vi "WPI_CANJaguar_SetPID.vi"(0 "CAN Jaguar Ref":T1={"DeviceStatus"={"status"=FALSE, "code"=0, "source"=""}, "Type"=enum."PWM", "PWM"={"PWM Channel"=enum."PWM 1", "DeadBand"={"Name"="", "maxPositivePwm"=0, "minPositivePwm"=0, "centerPwm"=0, "maxNegativePwm"=0, "minNegativePwm"=0, "angularRange"=0}}, "CAN"={"Device Number"=0, "Control Mode"=enum."Percent VBus", "Semaphore"=refnum, "Max Vout"=12.0, "TalonSRX Control Mode"=enum."Percent VBus"}, "Invert"=FALSE}, 5 "P":dbl, 7 "I":dbl, 9 "D":dbl, 11 "error in (no error)":errorcluster) -> (4 "CAN Jaguar Ref":T1={"DeviceStatus"={"status"=FALSE, "code"=0, "source"=""}, "Type"=enum."PWM", "PWM"={"PWM Channel"=enum."PWM 1", "DeadBand"={"Name"="", "maxPositivePwm"=0, "minPositivePwm"=0, "centerPwm"=0, "maxNegativePwm"=0, "minNegativePwm"=0, "angularRange"=0}}, "CAN"={"Device Number"=0, "Control Mode"=enum."Percent VBus", "Semaphore"=refnum, "Max Vout"=12.0, "TalonSRX Control Mode"=enum."Percent VBus"}, "Invert"=FALSE}, 15 "error out":errorcluster)   [LabVIEW 2016]
doc: "Set the PID constants that should be used by the active controller on the Jaguar.\n\nThis VI only applies in <B>Current</B>, <B>Position</B>, and <B>Speed</B> modes."
uses:
  <vilib>/Rock Robotics/WPI/MotorControl/WPI_MotorControlDeviceRef.ctl
  <vilib>/Rock Robotics/WPI/MotorControl/WPI_MotorControlType.ctl
  <vilib>/Rock Robotics/SystemInterfaces/DIO/FPGA_DIOPWMChannel.ctl
  <vilib>/Rock Robotics/WPI/PWM/WPI_PWMDeadband.ctl
  <vilib>/Rock Robotics/WPI/CAN/Jaguar/SubVIs/WPI_CANJaguar_ControlMode.ctl
  <vilib>/Rock Robotics/WPI/CAN/TalonSRX/WPI_CANTalonSRX_APIControlMode.ctl
  <vilib>/Rock Robotics/WPI/CAN/Jaguar/SubVIs/WPI_CAN_MotorMessageIDs.ctl
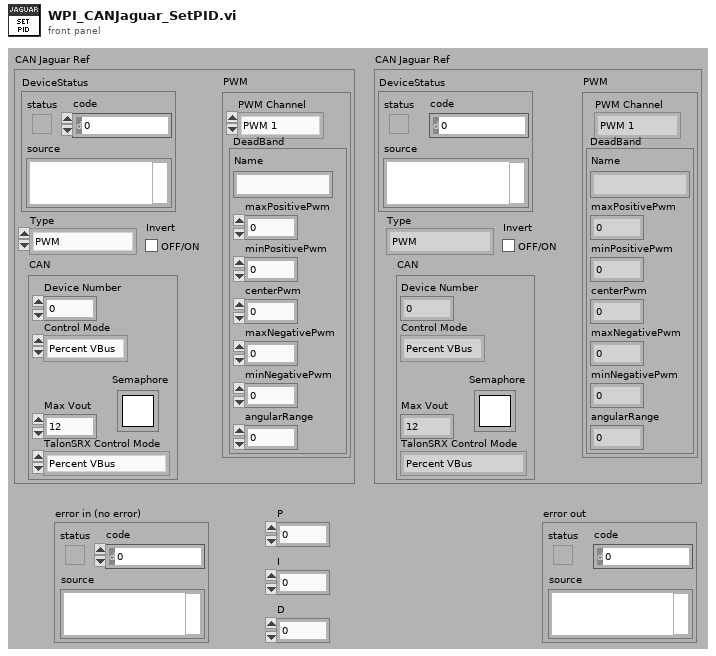
[diagram p1: front panel]
types:
  T1 = typedef "WPI_MotorControlDeviceRef.ctl" = cluster{"DeviceStatus":errorcluster, "Type":T2, "PWM":cluster{"PWM Channel":T3, "DeadBand":T4}, "CAN":cluster{"Device Number":u8, "Control Mode":T5, "Semaphore":T6, "Max Vout":dbl, "TalonSRX Control Mode":T7}, "Invert":bool}
  T2 = typedef "WPI_MotorControlType.ctl" = enum16{"PWM", "CAN", "CANTalonSRX"}
  T3 = typedef "FPGA_DIOPWMChannel.ctl" = enum8{"PWM 0", "PWM 1", "PWM 2", "PWM 3", "PWM 4", "PWM 5", "PWM 6", "PWM 7", "PWM 8", "PWM 9", "PWM MXP 0", "PWM MXP 1", "PWM MXP 2", "PWM MXP 3", "PWM MXP 4", "PWM MXP 5", "PWM MXP 6", "PWM MXP 7", "PWM MXP 8", "PWM MXP 9", "Invalid"}
  T4 = typedef "WPI_PWMDeadband.ctl" = cluster{"Name":string, "maxPositivePwm":i32, "minPositivePwm":i32, "centerPwm":i32, "maxNegativePwm":i32, "minNegativePwm":i32, "angularRange":u16}
  T5 = typedef "WPI_CANJaguar_ControlMode.ctl" = enum8{"Percent VBus", "Current", "Speed", "Position", "Voltage"}
  T6 = typedef "Semaphore RefNum" = refnum<k1>
  T7 = typedef "WPI_CANTalonSRX_APIControlMode.ctl" = enum8{"Percent VBus", "Speed", "Position", "Slave", "Unchanged / Invalid", "Voltage Compensation", "Current", "Motion Profile"}
  T8 = enum16{"big-endian, network order", "native, host order", "little-endian"}
  T9 = typedef "WPI_CAN_MotorMessageIDs.ctl" = u32
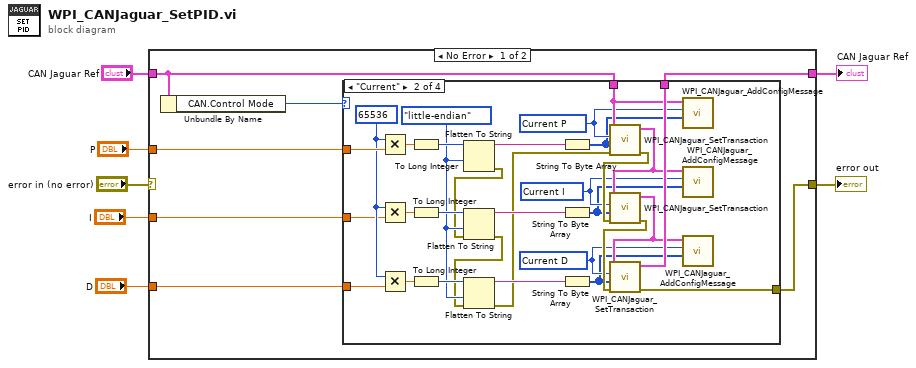
[diagram p0: block diagram]
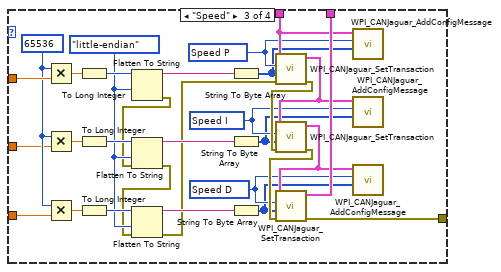
[diagram p3: hidden frame]
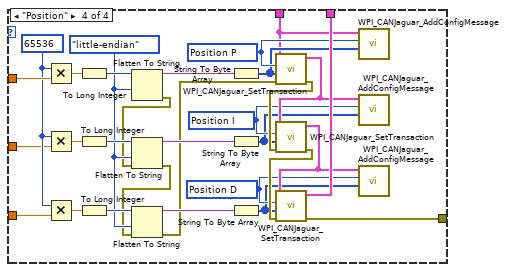
[diagram p4: hidden frame]
diagram:
  n1 = case shown="No Error" "error in (no error)" {
    selector: "error in (no error)" -> [_ w106]
    tunnel: [w11 w106] -> w7
    tunnel: [w8 w107] -> w5
    tunnel: "CAN Jaguar Ref" -> [w9 w107]
    tunnel: "P" -> [w14 _]
    tunnel: "D" -> [w13 _]
    tunnel: "I" -> [w12 _]
    frame No Error {
      n2 = Unbundle By Name(w9) -> ("CAN.Control Mode"=w10:T5)
      n3 = case shown="\"Current\"" w10 {
        tunnel: w14 -> [_ w43 w73 w103]
        tunnel: w13 -> [_ w33 w63 w93]
        tunnel: w12 -> [_ w32 w62 w92]
        tunnel: [_ w27 w58 w88] -> w11
        tunnel: w9 -> [w15 w24 w54 w82]
        tunnel: [w15 w28 w57 w87] -> w8
        frame Default {
        }
        frame "Current" {
          w35 = T8."little-endian" ("byte order (0:big-endian, network order)")
          w17 = T9 33689920 items=["Volt Enable"=33685504, "Volt Disable"=33685568, "Volt Set"=33685632, "Volt Set Ramp"=33685696, "Speed Enable"=33686528, "Speed Disable"=33686592, "Speed Set"=33686656, "Speed P"=33686720, "Speed I"=33686784, "Speed D"=33686848, "Speed Ref"=33686912, "Volt Comp Enable"=33687552, "Volt Comp Disable"=33687616, "Volt Comp Set"=33687680, "Volt Comp In Ramp"=33687744, "Volt Comp Comp Ramp"=33687808, "Position Enable"=33688576, "Position Disable"=33688640, "Position Set"=33688704, "Position P"=33688768, "Position I"=33688832, "Position D"=33688896, "Position Ref"=33688960, "Current Enable"=33689600, "Current Disable"=33689664, "Current Set"=33689728, "Current P"=33689792, "Current I"=33689856, "Current D"=33689920, "Status Percent VBus"=33690624, "Status VBus"=33690688, "Status Current"=33690752, "Status Temp"=33690816, "Status Position"=33690880, "Status Speed"=33690944, "Status Limit"=33691008, "Status Fault"=33691072, "Status Power"=33691136, "Status Control Mode"=33691200, "Status VOut"=33691264, "Config Num Brushes"=33692672, "Config Encoder Lines"=33692736, "Config Pot Turns"=33692800, "Config Brake Coast"=33692864, "Config Limit Mode"=33692928, "Config Limit Fwd"=33692992, "Config Limit Rev"=33693056, "Config Max VOut"=33693120, "Config Fault Time"=33693184, "Motor Ack"=33693696] ("CAN Motor Message IDs")
          w20 = T9 33689856 items=["Volt Enable"=33685504, "Volt Disable"=33685568, "Volt Set"=33685632, "Volt Set Ramp"=33685696, "Speed Enable"=33686528, "Speed Disable"=33686592, "Speed Set"=33686656, "Speed P"=33686720, "Speed I"=33686784, "Speed D"=33686848, "Speed Ref"=33686912, "Volt Comp Enable"=33687552, "Volt Comp Disable"=33687616, "Volt Comp Set"=33687680, "Volt Comp In Ramp"=33687744, "Volt Comp Comp Ramp"=33687808, "Position Enable"=33688576, "Position Disable"=33688640, "Position Set"=33688704, "Position P"=33688768, "Position I"=33688832, "Position D"=33688896, "Position Ref"=33688960, "Current Enable"=33689600, "Current Disable"=33689664, "Current Set"=33689728, "Current P"=33689792, "Current I"=33689856, "Current D"=33689920, "Status Percent VBus"=33690624, "Status VBus"=33690688, "Status Current"=33690752, "Status Temp"=33690816, "Status Position"=33690880, "Status Speed"=33690944, "Status Limit"=33691008, "Status Fault"=33691072, "Status Power"=33691136, "Status Control Mode"=33691200, "Status VOut"=33691264, "Config Num Brushes"=33692672, "Config Encoder Lines"=33692736, "Config Pot Turns"=33692800, "Config Brake Coast"=33692864, "Config Limit Mode"=33692928, "Config Limit Fwd"=33692992, "Config Limit Rev"=33693056, "Config Max VOut"=33693120, "Config Fault Time"=33693184, "Motor Ack"=33693696] ("CAN Motor Message IDs")
          w34 = 65536
          w23 = T9 33689792 items=["Volt Enable"=33685504, "Volt Disable"=33685568, "Volt Set"=33685632, "Volt Set Ramp"=33685696, "Speed Enable"=33686528, "Speed Disable"=33686592, "Speed Set"=33686656, "Speed P"=33686720, "Speed I"=33686784, "Speed D"=33686848, "Speed Ref"=33686912, "Volt Comp Enable"=33687552, "Volt Comp Disable"=33687616, "Volt Comp Set"=33687680, "Volt Comp In Ramp"=33687744, "Volt Comp Comp Ramp"=33687808, "Position Enable"=33688576, "Position Disable"=33688640, "Position Set"=33688704, "Position P"=33688768, "Position I"=33688832, "Position D"=33688896, "Position Ref"=33688960, "Current Enable"=33689600, "Current Disable"=33689664, "Current Set"=33689728, "Current P"=33689792, "Current I"=33689856, "Current D"=33689920, "Status Percent VBus"=33690624, "Status VBus"=33690688, "Status Current"=33690752, "Status Temp"=33690816, "Status Position"=33690880, "Status Speed"=33690944, "Status Limit"=33691008, "Status Fault"=33691072, "Status Power"=33691136, "Status Control Mode"=33691200, "Status VOut"=33691264, "Config Num Brushes"=33692672, "Config Encoder Lines"=33692736, "Config Pot Turns"=33692800, "Config Brake Coast"=33692864, "Config Limit Mode"=33692928, "Config Limit Fwd"=33692992, "Config Limit Rev"=33693056, "Config Max VOut"=33693120, "Config Fault Time"=33693184, "Motor Ack"=33693696] ("CAN Motor Message IDs")
          n4 = Multiply(x=w34, y=w43) -> (x*y=w44:dbl)
          n5 = Multiply(x=w34, y=w32) -> (x*y=w42:dbl)
          n6 = Multiply(x=w34, y=w33) -> (x*y=w39:dbl)
          n7 = To Long Integer(number=w44) -> (32bit integer=w45:i32)
          n8 = To Long Integer(number=w42) -> (32bit integer=w41:i32)
          n9 = To Long Integer(number=w39) -> (32bit integer=w40:i32)
          n10 = Flatten To String(anything=w45, byte order (0:big-endian, network order)=w35) -> (data string=w38:string, error out=w31:errorcluster)  [unwired: 1 in, 2 out]
          n11 = Flatten To String(anything=w41, byte order (0:big-endian, network order)=w35, error in (no error)=w31) -> (data string=w37:string, error out=w30:errorcluster)  [unwired: 2 out]
          n12 = Flatten To String(anything=w40, byte order (0:big-endian, network order)=w35, error in (no error)=w30) -> (data string=w36:string, error out=w29:errorcluster)  [unwired: 2 out]
          n13 = String To Byte Array(string=w38) -> (unsigned byte array=w22:u8[])
          n14 = String To Byte Array(string=w37) -> (unsigned byte array=w19:u8[])
          n15 = String To Byte Array(string=w36) -> (unsigned byte array=w16:u8[])
          n16 = call <vilib>:"WPI_CANJaguar_SetTransaction.vi"("error in"=w29, "Data"=w22, "Message ID"=w23, "CAN Jaguar Ref"=w24) -> ("error out"=w26:errorcluster, "CAN Jaguar Ref Out"=w21:T1)  [unwired: 6 out]
          n17 = call <vilib>:"WPI_CANJaguar_SetTransaction.vi"("error in"=w26, "Data"=w19, "Message ID"=w20, "CAN Jaguar Ref"=w21) -> ("error out"=w25:errorcluster, "CAN Jaguar Ref Out"=w18:T1)  [unwired: 6 out]
          n18 = call <vilib>:"WPI_CANJaguar_SetTransaction.vi"("error in"=w25, "Data"=w16, "Message ID"=w17, "CAN Jaguar Ref"=w18) -> ("error out"=w27:errorcluster, "CAN Jaguar Ref Out"=w28:T1)  [unwired: 6 out]
          n19 = call <vilib>:"WPI_CANJaguar_AddConfigMessage.vi"("Data"=w22, "Message ID"=w23, "CAN Jaguar Ref"=w24) -> ()  [unwired: 9 in]
          n20 = call <vilib>:"WPI_CANJaguar_AddConfigMessage.vi"("Data"=w19, "Message ID"=w20, "CAN Jaguar Ref"=w21) -> ()  [unwired: 9 in]
          n21 = call <vilib>:"WPI_CANJaguar_AddConfigMessage.vi"("Data"=w16, "Message ID"=w17, "CAN Jaguar Ref"=w18) -> ()  [unwired: 9 in]
        }
        frame "Speed" {
          w65 = T8."little-endian" ("byte order (0:big-endian, network order)")
          w47 = T9 33686848 items=["Volt Enable"=33685504, "Volt Disable"=33685568, "Volt Set"=33685632, "Volt Set Ramp"=33685696, "Speed Enable"=33686528, "Speed Disable"=33686592, "Speed Set"=33686656, "Speed P"=33686720, "Speed I"=33686784, "Speed D"=33686848, "Speed Ref"=33686912, "Volt Comp Enable"=33687552, "Volt Comp Disable"=33687616, "Volt Comp Set"=33687680, "Volt Comp In Ramp"=33687744, "Volt Comp Comp Ramp"=33687808, "Position Enable"=33688576, "Position Disable"=33688640, "Position Set"=33688704, "Position P"=33688768, "Position I"=33688832, "Position D"=33688896, "Position Ref"=33688960, "Current Enable"=33689600, "Current Disable"=33689664, "Current Set"=33689728, "Current P"=33689792, "Current I"=33689856, "Current D"=33689920, "Status Percent VBus"=33690624, "Status VBus"=33690688, "Status Current"=33690752, "Status Temp"=33690816, "Status Position"=33690880, "Status Speed"=33690944, "Status Limit"=33691008, "Status Fault"=33691072, "Status Power"=33691136, "Status Control Mode"=33691200, "Status VOut"=33691264, "Config Num Brushes"=33692672, "Config Encoder Lines"=33692736, "Config Pot Turns"=33692800, "Config Brake Coast"=33692864, "Config Limit Mode"=33692928, "Config Limit Fwd"=33692992, "Config Limit Rev"=33693056, "Config Max VOut"=33693120, "Config Fault Time"=33693184, "Motor Ack"=33693696] ("CAN Motor Message IDs")
          w50 = T9 33686784 items=["Volt Enable"=33685504, "Volt Disable"=33685568, "Volt Set"=33685632, "Volt Set Ramp"=33685696, "Speed Enable"=33686528, "Speed Disable"=33686592, "Speed Set"=33686656, "Speed P"=33686720, "Speed I"=33686784, "Speed D"=33686848, "Speed Ref"=33686912, "Volt Comp Enable"=33687552, "Volt Comp Disable"=33687616, "Volt Comp Set"=33687680, "Volt Comp In Ramp"=33687744, "Volt Comp Comp Ramp"=33687808, "Position Enable"=33688576, "Position Disable"=33688640, "Position Set"=33688704, "Position P"=33688768, "Position I"=33688832, "Position D"=33688896, "Position Ref"=33688960, "Current Enable"=33689600, "Current Disable"=33689664, "Current Set"=33689728, "Current P"=33689792, "Current I"=33689856, "Current D"=33689920, "Status Percent VBus"=33690624, "Status VBus"=33690688, "Status Current"=33690752, "Status Temp"=33690816, "Status Position"=33690880, "Status Speed"=33690944, "Status Limit"=33691008, "Status Fault"=33691072, "Status Power"=33691136, "Status Control Mode"=33691200, "Status VOut"=33691264, "Config Num Brushes"=33692672, "Config Encoder Lines"=33692736, "Config Pot Turns"=33692800, "Config Brake Coast"=33692864, "Config Limit Mode"=33692928, "Config Limit Fwd"=33692992, "Config Limit Rev"=33693056, "Config Max VOut"=33693120, "Config Fault Time"=33693184, "Motor Ack"=33693696] ("CAN Motor Message IDs")
          w64 = 65536
          w53 = T9 33686720 items=["Volt Enable"=33685504, "Volt Disable"=33685568, "Volt Set"=33685632, "Volt Set Ramp"=33685696, "Speed Enable"=33686528, "Speed Disable"=33686592, "Speed Set"=33686656, "Speed P"=33686720, "Speed I"=33686784, "Speed D"=33686848, "Speed Ref"=33686912, "Volt Comp Enable"=33687552, "Volt Comp Disable"=33687616, "Volt Comp Set"=33687680, "Volt Comp In Ramp"=33687744, "Volt Comp Comp Ramp"=33687808, "Position Enable"=33688576, "Position Disable"=33688640, "Position Set"=33688704, "Position P"=33688768, "Position I"=33688832, "Position D"=33688896, "Position Ref"=33688960, "Current Enable"=33689600, "Current Disable"=33689664, "Current Set"=33689728, "Current P"=33689792, "Current I"=33689856, "Current D"=33689920, "Status Percent VBus"=33690624, "Status VBus"=33690688, "Status Current"=33690752, "Status Temp"=33690816, "Status Position"=33690880, "Status Speed"=33690944, "Status Limit"=33691008, "Status Fault"=33691072, "Status Power"=33691136, "Status Control Mode"=33691200, "Status VOut"=33691264, "Config Num Brushes"=33692672, "Config Encoder Lines"=33692736, "Config Pot Turns"=33692800, "Config Brake Coast"=33692864, "Config Limit Mode"=33692928, "Config Limit Fwd"=33692992, "Config Limit Rev"=33693056, "Config Max VOut"=33693120, "Config Fault Time"=33693184, "Motor Ack"=33693696] ("CAN Motor Message IDs")
          n22 = Multiply(x=w64, y=w73) -> (x*y=w74:dbl)
          n23 = Multiply(x=w64, y=w62) -> (x*y=w72:dbl)
          n24 = Multiply(x=w64, y=w63) -> (x*y=w69:dbl)
          n25 = To Long Integer(number=w74) -> (32bit integer=w75:i32)
          n26 = To Long Integer(number=w72) -> (32bit integer=w71:i32)
          n27 = To Long Integer(number=w69) -> (32bit integer=w70:i32)
          n28 = Flatten To String(anything=w75, byte order (0:big-endian, network order)=w65) -> (data string=w68:string, error out=w61:errorcluster)  [unwired: 1 in, 2 out]
          n29 = Flatten To String(anything=w71, byte order (0:big-endian, network order)=w65, error in (no error)=w61) -> (data string=w67:string, error out=w60:errorcluster)  [unwired: 2 out]
          n30 = Flatten To String(anything=w70, byte order (0:big-endian, network order)=w65, error in (no error)=w60) -> (data string=w66:string, error out=w59:errorcluster)  [unwired: 2 out]
          n31 = String To Byte Array(string=w68) -> (unsigned byte array=w52:u8[])
          n32 = String To Byte Array(string=w67) -> (unsigned byte array=w49:u8[])
          n33 = String To Byte Array(string=w66) -> (unsigned byte array=w46:u8[])
          n34 = call <vilib>:"WPI_CANJaguar_SetTransaction.vi"("error in"=w59, "Data"=w52, "Message ID"=w53, "CAN Jaguar Ref"=w54) -> ("error out"=w56:errorcluster, "CAN Jaguar Ref Out"=w51:T1)  [unwired: 6 out]
          n35 = call <vilib>:"WPI_CANJaguar_SetTransaction.vi"("error in"=w56, "Data"=w49, "Message ID"=w50, "CAN Jaguar Ref"=w51) -> ("error out"=w55:errorcluster, "CAN Jaguar Ref Out"=w48:T1)  [unwired: 6 out]
          n36 = call <vilib>:"WPI_CANJaguar_SetTransaction.vi"("error in"=w55, "Data"=w46, "Message ID"=w47, "CAN Jaguar Ref"=w48) -> ("error out"=w58:errorcluster, "CAN Jaguar Ref Out"=w57:T1)  [unwired: 6 out]
          n37 = call <vilib>:"WPI_CANJaguar_AddConfigMessage.vi"("Data"=w52, "Message ID"=w53, "CAN Jaguar Ref"=w54) -> ()  [unwired: 9 in]
          n38 = call <vilib>:"WPI_CANJaguar_AddConfigMessage.vi"("Data"=w49, "Message ID"=w50, "CAN Jaguar Ref"=w51) -> ()  [unwired: 9 in]
          n39 = call <vilib>:"WPI_CANJaguar_AddConfigMessage.vi"("Data"=w46, "Message ID"=w47, "CAN Jaguar Ref"=w48) -> ()  [unwired: 9 in]
        }
        frame "Position" {
          w95 = T8."little-endian" ("byte order (0:big-endian, network order)")
          w77 = T9 33688896 items=["Volt Enable"=33685504, "Volt Disable"=33685568, "Volt Set"=33685632, "Volt Set Ramp"=33685696, "Speed Enable"=33686528, "Speed Disable"=33686592, "Speed Set"=33686656, "Speed P"=33686720, "Speed I"=33686784, "Speed D"=33686848, "Speed Ref"=33686912, "Volt Comp Enable"=33687552, "Volt Comp Disable"=33687616, "Volt Comp Set"=33687680, "Volt Comp In Ramp"=33687744, "Volt Comp Comp Ramp"=33687808, "Position Enable"=33688576, "Position Disable"=33688640, "Position Set"=33688704, "Position P"=33688768, "Position I"=33688832, "Position D"=33688896, "Position Ref"=33688960, "Current Enable"=33689600, "Current Disable"=33689664, "Current Set"=33689728, "Current P"=33689792, "Current I"=33689856, "Current D"=33689920, "Status Percent VBus"=33690624, "Status VBus"=33690688, "Status Current"=33690752, "Status Temp"=33690816, "Status Position"=33690880, "Status Speed"=33690944, "Status Limit"=33691008, "Status Fault"=33691072, "Status Power"=33691136, "Status Control Mode"=33691200, "Status VOut"=33691264, "Config Num Brushes"=33692672, "Config Encoder Lines"=33692736, "Config Pot Turns"=33692800, "Config Brake Coast"=33692864, "Config Limit Mode"=33692928, "Config Limit Fwd"=33692992, "Config Limit Rev"=33693056, "Config Max VOut"=33693120, "Config Fault Time"=33693184, "Motor Ack"=33693696] ("CAN Motor Message IDs")
          w80 = T9 33688832 items=["Volt Enable"=33685504, "Volt Disable"=33685568, "Volt Set"=33685632, "Volt Set Ramp"=33685696, "Speed Enable"=33686528, "Speed Disable"=33686592, "Speed Set"=33686656, "Speed P"=33686720, "Speed I"=33686784, "Speed D"=33686848, "Speed Ref"=33686912, "Volt Comp Enable"=33687552, "Volt Comp Disable"=33687616, "Volt Comp Set"=33687680, "Volt Comp In Ramp"=33687744, "Volt Comp Comp Ramp"=33687808, "Position Enable"=33688576, "Position Disable"=33688640, "Position Set"=33688704, "Position P"=33688768, "Position I"=33688832, "Position D"=33688896, "Position Ref"=33688960, "Current Enable"=33689600, "Current Disable"=33689664, "Current Set"=33689728, "Current P"=33689792, "Current I"=33689856, "Current D"=33689920, "Status Percent VBus"=33690624, "Status VBus"=33690688, "Status Current"=33690752, "Status Temp"=33690816, "Status Position"=33690880, "Status Speed"=33690944, "Status Limit"=33691008, "Status Fault"=33691072, "Status Power"=33691136, "Status Control Mode"=33691200, "Status VOut"=33691264, "Config Num Brushes"=33692672, "Config Encoder Lines"=33692736, "Config Pot Turns"=33692800, "Config Brake Coast"=33692864, "Config Limit Mode"=33692928, "Config Limit Fwd"=33692992, "Config Limit Rev"=33693056, "Config Max VOut"=33693120, "Config Fault Time"=33693184, "Motor Ack"=33693696] ("CAN Motor Message IDs")
          w94 = 65536
          w84 = T9 33688768 items=["Volt Enable"=33685504, "Volt Disable"=33685568, "Volt Set"=33685632, "Volt Set Ramp"=33685696, "Speed Enable"=33686528, "Speed Disable"=33686592, "Speed Set"=33686656, "Speed P"=33686720, "Speed I"=33686784, "Speed D"=33686848, "Speed Ref"=33686912, "Volt Comp Enable"=33687552, "Volt Comp Disable"=33687616, "Volt Comp Set"=33687680, "Volt Comp In Ramp"=33687744, "Volt Comp Comp Ramp"=33687808, "Position Enable"=33688576, "Position Disable"=33688640, "Position Set"=33688704, "Position P"=33688768, "Position I"=33688832, "Position D"=33688896, "Position Ref"=33688960, "Current Enable"=33689600, "Current Disable"=33689664, "Current Set"=33689728, "Current P"=33689792, "Current I"=33689856, "Current D"=33689920, "Status Percent VBus"=33690624, "Status VBus"=33690688, "Status Current"=33690752, "Status Temp"=33690816, "Status Position"=33690880, "Status Speed"=33690944, "Status Limit"=33691008, "Status Fault"=33691072, "Status Power"=33691136, "Status Control Mode"=33691200, "Status VOut"=33691264, "Config Num Brushes"=33692672, "Config Encoder Lines"=33692736, "Config Pot Turns"=33692800, "Config Brake Coast"=33692864, "Config Limit Mode"=33692928, "Config Limit Fwd"=33692992, "Config Limit Rev"=33693056, "Config Max VOut"=33693120, "Config Fault Time"=33693184, "Motor Ack"=33693696] ("CAN Motor Message IDs")
          n40 = Multiply(x=w94, y=w103) -> (x*y=w104:dbl)
          n41 = Multiply(x=w94, y=w92) -> (x*y=w102:dbl)
          n42 = Multiply(x=w94, y=w93) -> (x*y=w99:dbl)
          n43 = To Long Integer(number=w104) -> (32bit integer=w105:i32)
          n44 = To Long Integer(number=w102) -> (32bit integer=w101:i32)
          n45 = To Long Integer(number=w99) -> (32bit integer=w100:i32)
          n46 = Flatten To String(anything=w105, byte order (0:big-endian, network order)=w95) -> (data string=w98:string, error out=w91:errorcluster)  [unwired: 1 in, 2 out]
          n47 = Flatten To String(anything=w101, byte order (0:big-endian, network order)=w95, error in (no error)=w91) -> (data string=w97:string, error out=w90:errorcluster)  [unwired: 2 out]
          n48 = Flatten To String(anything=w100, byte order (0:big-endian, network order)=w95, error in (no error)=w90) -> (data string=w96:string, error out=w89:errorcluster)  [unwired: 2 out]
          n49 = String To Byte Array(string=w98) -> (unsigned byte array=w83:u8[])
          n50 = String To Byte Array(string=w97) -> (unsigned byte array=w79:u8[])
          n51 = String To Byte Array(string=w96) -> (unsigned byte array=w76:u8[])
          n52 = call <vilib>:"WPI_CANJaguar_SetTransaction.vi"("error in"=w89, "Data"=w83, "Message ID"=w84, "CAN Jaguar Ref"=w82) -> ("error out"=w86:errorcluster, "CAN Jaguar Ref Out"=w81:T1)  [unwired: 6 out]
          n53 = call <vilib>:"WPI_CANJaguar_SetTransaction.vi"("error in"=w86, "Data"=w79, "Message ID"=w80, "CAN Jaguar Ref"=w81) -> ("error out"=w85:errorcluster, "CAN Jaguar Ref Out"=w78:T1)  [unwired: 6 out]
          n54 = call <vilib>:"WPI_CANJaguar_SetTransaction.vi"("error in"=w85, "Data"=w76, "Message ID"=w77, "CAN Jaguar Ref"=w78) -> ("error out"=w88:errorcluster, "CAN Jaguar Ref Out"=w87:T1)  [unwired: 6 out]
          n55 = call <vilib>:"WPI_CANJaguar_AddConfigMessage.vi"("Data"=w83, "Message ID"=w84, "CAN Jaguar Ref"=w82) -> ()  [unwired: 9 in]
          n56 = call <vilib>:"WPI_CANJaguar_AddConfigMessage.vi"("Data"=w79, "Message ID"=w80, "CAN Jaguar Ref"=w81) -> ()  [unwired: 9 in]
          n57 = call <vilib>:"WPI_CANJaguar_AddConfigMessage.vi"("Data"=w76, "Message ID"=w77, "CAN Jaguar Ref"=w78) -> ()  [unwired: 9 in]
        }
      }
    }
    frame Error {
    }
  }
  "CAN Jaguar Ref" <- w5
  "error out" <- w7
